vi "BRig_dataTrial_n_ENL.vi"() -> (2 "output_ENL_n":i32)   [LabVIEW 2014]
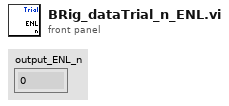
[diagram p1: front panel]
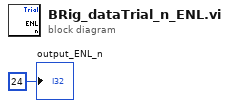
[diagram p0: block diagram]
diagram:
  "output_ENL_n" <- 24 ("output_iBlock")
